vi "DownloadString.vi"(4 "File":T1, 6 "error in":errorcluster) -> (0 "error out":errorcluster, 3 "file":string)   [LabVIEW 2014, in "Raspberry Pi Compatible Compiler for LabVIEW.lvlib" / "GitHub API.lvlib"]
uses:
  GitHub API.lvlib
  TypeDefs/GitHubContents_TD.ctl
  <vilib>/httpClient/LabVIEWHTTPClient.lvlib
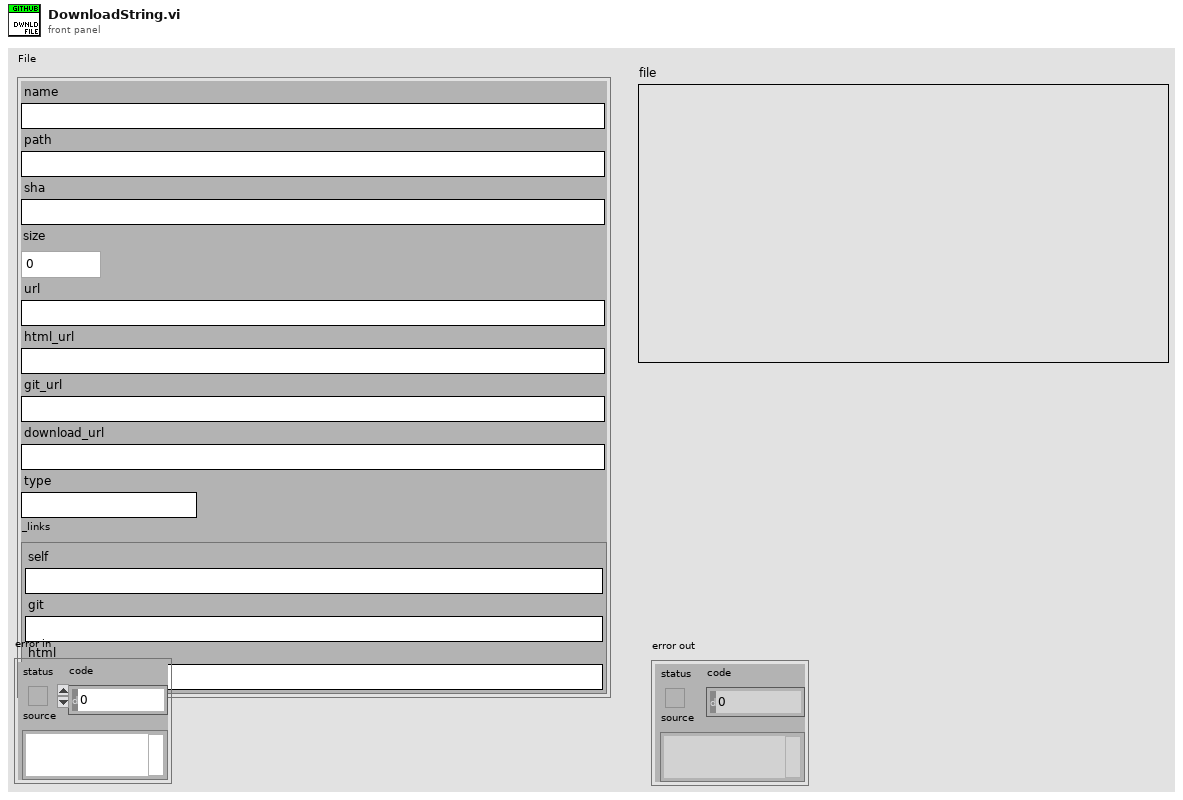
[diagram p1: front panel]
types:
  T1 = typedef "Raspberry Pi Compatible Compiler for LabVIEW.lvlib/GitHub API.lvlib/GitHubContents_TD.ctl" = cluster{"name":string, "path":string, "sha":string, "size":dbl, "url":string, "html_url":string, "git_url":string, "download_url":string, "type":string, "_links":cluster{"self":string, "git":string, "html":string}}
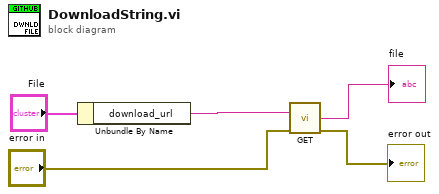
[diagram p0: block diagram]
diagram:
  n1 = Unbundle By Name("File") -> ("download_url"=w4:string)
  n2 = call <vilib>:"GET.vi"("url"=w4, "error in (no error)"="error in") -> ("body"=→"file":string, "error out"=→"error out":errorcluster)  [unwired: 10 in, 2 out]
